vi "CANSendMotorSpeed.vi"(7 "Remote":bool=TRUE, 8 "error in (no error)":errorcluster, 9 "Motor Speed RPM":u16, 10 "UUT":refnum<vi>, 11 "CAN Cluster in":refnum<vi>) -> (0 "error out":errorcluster caption="错误输出")   [LabVIEW 2017]
uses:
  Marvin CAN Bus 21.5.18/PCAN_Driver/ControlCAN.llb/VCI_CAN_OBJ.ctl
  PCAN_Driver/ControlCAN.lvlib
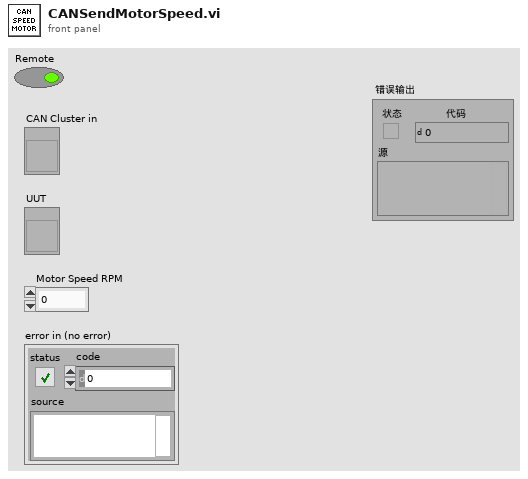
[diagram p1: front panel]
types:
  T1 = typedef "ControlCAN.lvlib/VCI_CAN_OBJ.ctl" = cluster{"ID":u32, "TimeStamp":u32, "TimeFlag":u8, "SendType":u8, "RemoteFlag":u8, "ExternFlag":u8, "DataLen":u8, "Data":u8[], "Reserved":u8[]}
  T2 = cluster{"ID":u32, "MSGTYPE":u8, "LEN":u8, "aDATA":u8[]}
  T3 = typedef "ControlCAN.lvlib/DevType.ctl" = u32
  T4 = typedef "ControlCAN.lvlib/CAN Channel.ctl" = u32
  T5 = typedef "ControlCAN.lvlib/VCI_INIT_CONFIG.ctl" = cluster{"AccCode":u32, "AccMask":u32, "InitFlag":T6, "Fliter":T7, "Timing0":u8, "Timing1":u8, "Mode":T8}
  T6 = typedef "ControlCAN.lvlib/InitFlag.ctl" = u32
  T7 = typedef "ControlCAN.lvlib/Fliter.ctl" = u8
  T8 = typedef "ControlCAN.lvlib/Mode.ctl" = u8
  T9 = cluster{"DevType":T3, "DevIndex":u32, "CanIndex":T4, "VCI_INIT_CONFIG":T5}
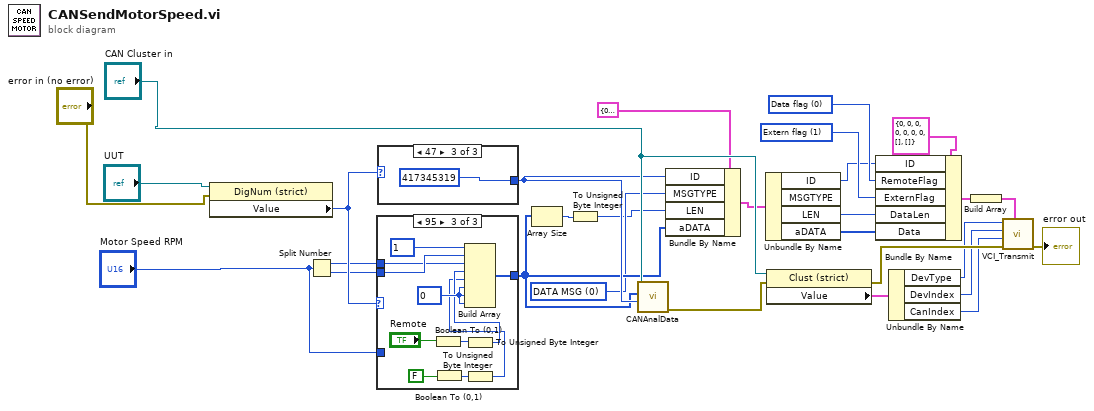
[diagram p0: block diagram]
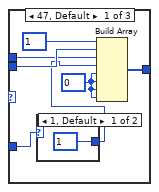
[diagram p2: hidden frame]
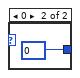
[diagram p3: hidden frame]
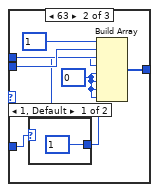
[diagram p4: hidden frame]
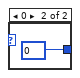
[diagram p5: hidden frame]
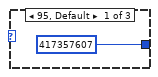
[diagram p6: hidden frame]
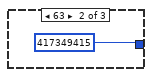
[diagram p7: hidden frame]
diagram:
  w17 = u8 0 items=["STATUS"=128, "EXTENDED"=2, "RTR"=1, "DATA MSG"=0] ("MSGTYPE")
  w12 = u8 1 items=["Standart flag", "Extern flag"] ("Format")
  w13 = u8 0 items=["Data flag", "Remote flag"] ("Type")
  n1 = property on="Property Node" class="DigNum (strict)"(reference="UUT", error in="error in (no error)") -> ("Value"=w23:u8)  [unwired: 2 out]
  n2 = Split Number(x="Motor Speed RPM") -> (hi(x)=w21:u8, lo(x)=w20:u8)
  n3 = case shown="95" w23 {
    tunnel: [w36 w45 w58] -> w19
    tunnel: w20 -> [w35 w44 w57]
    tunnel: w21 -> [w34 w43 w56]
    tunnel: "Motor Speed RPM" -> [w31 w40 _]
    frame 47, Default {
      w33 = u8 0 ("element")
      n4 = case shown="1, Default" w31 {
        tunnel: [u8 1 ("element") u8 0 ("element")] -> w30
        frame 1, Default {
        }
        frame 0 {
        }
      }
      n5 = Build Array(u8 1 ("element"), w35, w34, w30, w33, w33, w33, w33) -> (w36:u8[])
    }
    frame 63 {
      w41 = u8 0 ("element")
      n6 = case shown="1, Default" w40 {
        tunnel: [u8 1 ("element") u8 0 ("element")] -> w39
        frame 1, Default {
        }
        frame 0 {
        }
      }
      n7 = Build Array(u8 1 ("element"), w44, w43, w39, w41, w41, w41, w41) -> (w45:u8[])
    }
    frame 95 {
      w54 = u8 0 ("element")
      n8 = Boolean To (0,1)(Boolean="Remote") -> (0, 1=w52:i16)
      n9 = Boolean To (0,1)(Boolean=FALSE ("Motor Over Temp 2")) -> (0, 1=w53:i16)
      n10 = To Unsigned Byte Integer(number=w52) -> (unsigned 8bit integer=w50:u8)
      n11 = To Unsigned Byte Integer(number=w53) -> (unsigned 8bit integer=w49:u8)
      n12 = Build Array(u8 1 ("element"), w57, w56, w50, w49, w54, w54, w54) -> (w58:u8[])
    }
  }
  n13 = case shown="47" w23 {
    tunnel: [u32 417357607 u32 417349415 u32 417345319] -> w22
    frame 95, Default {
    }
    frame 63 {
    }
    frame 47 {
    }
  }
  n14 = Array Size(array=w19) -> (size(s)=w14:i32)
  n15 = To Unsigned Byte Integer(number=w14) -> (unsigned 8bit integer=w16:u8)
  n16 = call "CANAnalData.vi"("ID"=w22, "Data"=w19, "Config"="CAN Cluster in") -> ("error out"=w29:errorcluster)  [unwired: 4 in, 4 out]
  n17 = Bundle By Name(cluster=T2 {"ID"=0, "MSGTYPE"=0, "LEN"=0, "aDATA"=[]} ("MsgTX 2"), "ID"=w22, "MSGTYPE"=w17, "LEN"=w16, "aDATA"=w19) -> (w18:T2)
  n18 = Unbundle By Name(w18) -> ("ID"=w4:u32, "LEN"=w3:u8, "aDATA"=w2:u8[])  [unwired: 1 out]
  n19 = property class="Clust (strict)"(reference="CAN Cluster in", error in=w29) -> (error out=w28:errorcluster, "Value"=w5:T9)  [unwired: 1 out]
  n20 = Bundle By Name(cluster=T1 {"ID"=0, "TimeStamp"=0, "TimeFlag"=0, "SendType"=0, "RemoteFlag"=0, "ExternFlag"=0, "DataLen"=0, "Data"=[], "Reserved"=[]} ("Send"), "ID"=w4, "RemoteFlag"=w13, "ExternFlag"=w12, "DataLen"=w3, "Data"=w2) -> (w7:T1)
  n21 = Unbundle By Name(w5) -> ("DevType"=w11:T3, "DevIndex"=w10:u32, "CanIndex"=w9:T4)
  n22 = Build Array(w7) -> (w8:T1[])
  n23 = call "VCI_Transmit.vi"("Buffer"=w8, "error in (no error)"=w28, "CANIndex"=w9, "DevIndex"=w10, "DevType"=w11) -> ("error out"=→"error out":errorcluster)  [unwired: 6 out]
